vi "CRC_16_8.vi"() -> ()   [LabVIEW 2016]
panel:
  in  "data":u8[](array[numeric])
  out "CRC":u16 format="%x"
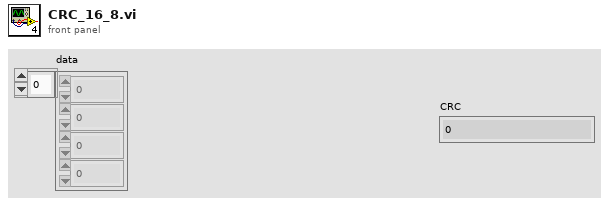
[diagram p1: front panel]
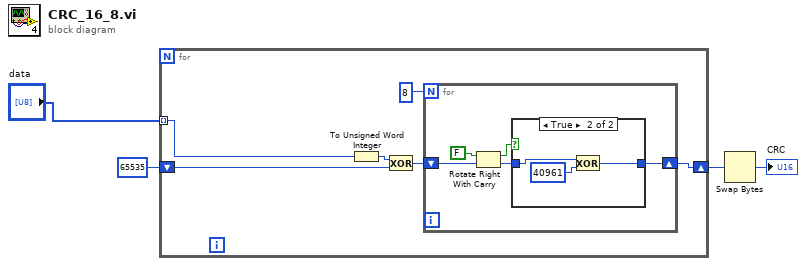
[diagram p0: block diagram]
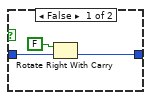
[diagram p2: hidden frame]
diagram:
  n1 = for {
    shift-right: [w7] -> w3
    shift-left: u16 65535 -> [w9]
    tunnel: "data" -> [w5] mode=indexing
    n2 = To Unsigned Word Integer(number=w5) -> (unsigned 16bit integer=w10:u16)
    n3 = Exclusive Or(1:w9, 2:w10) -> (0:w8:u16)
    n4 = for {
      N: 8 -> [_]
      shift-right: [w12] -> w7
      shift-left: w8 -> [w15]
      n5 = Rotate Right With Carry(2:w15, 3:FALSE) -> (0:w11:u16, 1:w13:bool)
      n6 = case shown="True" w13 {
        tunnel: w11 -> [w17 w21]
        tunnel: [w16 w19] -> w12
        frame False {
          n7 = Rotate Right With Carry(2:w17, 3:FALSE) -> (0:w16:u16)  [unwired: 1 out]
        }
        frame True {
          n8 = Exclusive Or(1:u16 40961 ("y"), 2:w21) -> (0:w19:u16)
        }
      }
    }
  }
  n9 = Swap Bytes(anything=w3) -> (byte swapped=→"CRC":u16)
